vi "Get SHA-1 Test Manager.vi"(8 "error in (no error)":errorcluster, 10 "Properties":refnum<class "Properties.lvclass">) -> (0 "error out":errorcluster, 1 "SHA-1 hash":string, 2 "Properties":refnum<class "Properties.lvclass">)   [LabVIEW 2021, in "Banana.Caraya.lvlib" / "Properties.Banana.lvclass"]
uses:
  Properties.Banana.lvclass
  <vilib>/addons/_JKI Toolkits/Caraya/classes/Properties/Properties.lvclass
  <vilib>/addons/_JKI Toolkits/Caraya/classes/Properties/Properties.lvclass/Properties.ctl
  <vilib>/LabVIEW Open Source Project/Cryptographic Functions/SHA-1/SHA-1.vi
  <vilib>/LabVIEW Open Source Project/Cryptographic Functions/SHA-1/SHA-1.lvclass
  Properties.Banana.lvclass/Properties.Banana.ctl
  <vilib>/LabVIEW Open Source Project/Cryptographic Functions/SHA-1/SHA-1.lvlib
  <vilib>/addons/_JKI Toolkits/Caraya/classes/Basic Test Manager/Basic Test Manager.lvclass
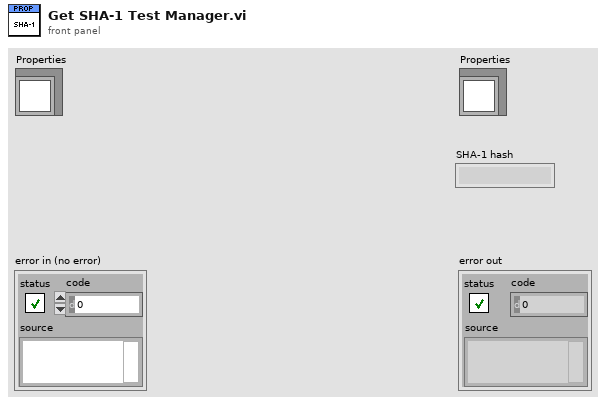
[diagram p1: front panel]
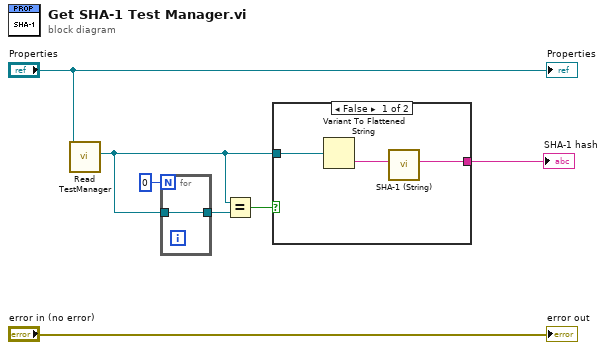
[diagram p0: block diagram]
diagram:
  n1 = call <vilib>:"Read TestManager.vi"("Properties in"="Properties") -> ("Test Manager"=w2:refnum<class "Basic Test Manager.lvclass">)  [unwired: 9 in, 1 out]
  n2 = for {
    N: 0 -> [_]
    tunnel: [w8] -> w3
    tunnel: w2 -> [w8]
  }
  n3 = Equal?(x=w2, y=w3) -> (x = y?=w4:bool)
  n4 = case shown="False" w4 {
    tunnel: [w11 _] -> w5
    tunnel: w2 -> [w9 _]
    frame False {
      n5 = Variant To Flattened String(Variant=w9) -> (data string=w10:string)  [unwired: 1 out]
      n6 = call <vilib>:"SHA-1 (String).vi"("message"=w10) -> ("SHA-1 hash"=w11:string)  [unwired: 10 in]
    }
    frame True {
    }
  }
  "SHA-1 hash" <- w5
  "error out" <- "error in (no error)"
  "Properties" <- "Properties"
